vi "Get State.vi"(8 "error in (no error)":errorcluster, 11 "Device in":refnum<class "Device.lvclass">) -> (0 "error out":errorcluster, 2 "Device State":T1, 3 "Device out":refnum<class "Device.lvclass">)   [LabVIEW 2020, in "HAL.lvlib" / "Device.lvclass"]
uses:
  Device.lvclass
  Device State.ctl
  Device.lvclass/Device.ctl
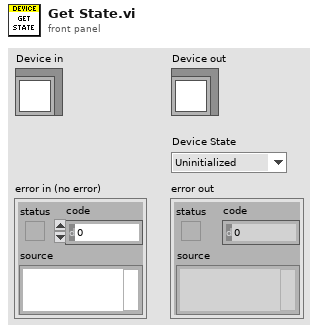
[diagram p1: front panel]
types:
  T1 = typedef "HAL.lvlib/Device.lvclass/Device State.ctl" = enum16{"Uninitialized", "Initialized", "Configured", "Running", "Error"}
  T2 = typedef "HAL.lvlib/Device.lvclass/Ref Data.ctl" = cluster{"Config Keys":string[], "Config Values":string[], "Cal Expires":timestamp, "Name":string, "Comment":string, "State":T1, "Error":errorcluster}
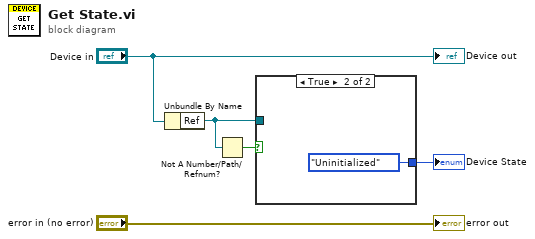
[diagram p0: block diagram]
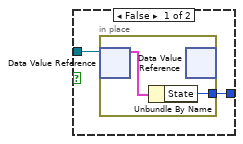
[diagram p2: hidden frame]
diagram:
  n1 = Unbundle By Name("Device in") -> ("Ref"=w2:refnum<data-value>)
  n2 = Not A Number/Path/Refnum?(number/path/refnum=w2) -> (NaN/Path/Refnum?=w1:bool)
  n3 = case shown="True" w1 {
    tunnel: [w7 Device_State."Uninitialized" ("State")] -> w3
    tunnel: w2 -> [w6 _]
    frame False {
      n4 = in-place {
        in-place-border: [w8] -> w7
        n5 = in-place-dvr #1(w6) -> (w9:T2)  [unwired: 1 out]
        n6 = Unbundle By Name(w9) -> ("State"=w8:T1)
        n7 = in-place-dvr #1() -> ()  [unwired: 1 in, 2 out]
      }
    }
    frame True {
    }
  }
  "Device State" <- w3
  "error out" <- "error in (no error)"
  "Device out" <- "Device in"
